vi "CRYSmoothing Waveform.vi"(8 "Weight Mode":u16(ring) items=["None", "Hanning"], 9 "Width (s)":dbl, 11 "Wave In":T1={"Waveform"={"X0"=0.0, "dX"=0.0, "Y"=[]}, "X data"=1, "Y data"=1, "Y axis"=1, "X unit"="s", "Y unit"="V", "Y dB ref"=1.0, "display Y"=TRUE, "display X"=TRUE, "Overload?"=FALSE, "Test Info"="", "Step No."=0, "Name"="", "protected"=FALSE, "Sqc history"=[], "Signal Channel ID"=0, "Plot Settings"={"Color"=0, "Interpolation"=0, "Point Style"=0, "Line Style"=0, "Point Color"=0, "Line Width"=0, "Bar Plot Style"=0, "Fill To"=0}, "AutoProtect"=FALSE} {"Y dB ref" format="%.1f"; "Y axis" items=["Log", "Lin"]; "Y data" items=["dB", "Lin"]; "X data" items=["dB", "Lin"]}) -> (3 "Wave out":T1={"Waveform"={"X0"=0.0, "dX"=0.0, "Y"=[]}, "X data"=1, "Y data"=1, "Y axis"=1, "X unit"="s", "Y unit"="V", "Y dB ref"=1.0, "display Y"=TRUE, "display X"=TRUE, "Overload?"=FALSE, "Test Info"="", "Step No."=0, "Name"="", "protected"=FALSE, "Sqc history"=[], "Signal Channel ID"=0, "Plot Settings"={"Color"=0, "Interpolation"=0, "Point Style"=0, "Line Style"=0, "Point Color"=0, "Line Width"=0, "Bar Plot Style"=0, "Fill To"=0}, "AutoProtect"=FALSE} {"Y dB ref" format="%.1f"; "Y axis" items=["Log", "Lin"]; "Y data" items=["dB", "Lin"]; "X data" items=["dB", "Lin"]})   [LabVIEW 2013]
uses:
  Typedef Control/CRYWaveform Cluster.ctl
  <vilib>/Analysis/2dsp.llb/1D Convolution (DBL).vi
  <vilib>/Analysis/0measdsp.llb/Scaled Time Domain Window (DBL).vi
  <vilib>/Analysis/NI_AALPro.lvlib
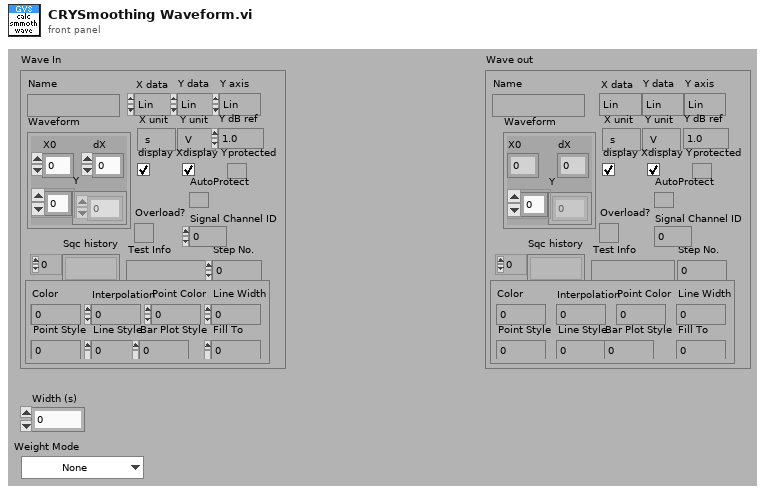
[diagram p1: front panel]
types:
  T1 = typedef "CRYWaveform Cluster.ctl" = cluster{"Waveform":cluster{"X0":dbl, "dX":dbl, "Y":sgl[]}, "X data":u16, "Y data":u16, "Y axis":u16, "X unit":string, "Y unit":string, "Y dB ref":dbl, "display Y":bool, "display X":bool, "Overload?":bool, "Test Info":string, "Step No.":i32, "Name":string, "protected":bool, "Sqc history":string[], "Signal Channel ID":i32, "Plot Settings":cluster{"Color":u32, "Interpolation":u8, "Point Style":u8, "Line Style":u8, "Point Color":u32, "Line Width":u8, "Bar Plot Style":u8, "Fill To":i16}, "AutoProtect":bool}
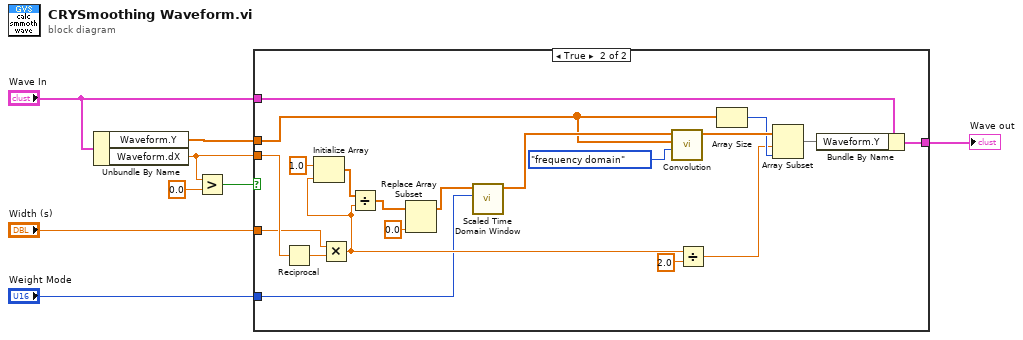
[diagram p0: block diagram]
diagram:
  n1 = Unbundle By Name("Wave In") -> ("Waveform.Y"=w8:sgl[], "Waveform.dX"=w1:dbl)
  n2 = Greater?(x=w1, y=0.0) -> (0:w2:bool)
  n3 = case shown="True" w2 {
    tunnel: w8 -> [_ w17]
    tunnel: w1 -> [_ w15]
    tunnel: "Wave In" -> [w9 w13]
    tunnel: "Width (s)" -> [_ w12]
    tunnel: "Weight Mode" -> [_ w11]
    tunnel: [w9 w10] -> w4
    frame False {
    }
    frame True {
      n4 = Reciprocal(x=w15) -> (1/x=w14:dbl)
      n5 = Multiply(x=w12, y=w14) -> (x*y=w20:dbl)
      n6 = Initialize Array(1.0 ("element"), w20) -> (w28:dbl[])
      n7 = Divide(x=w28, y=w20) -> (x/y=w25:dbl[])
      n8 = Replace Array Subset(array=w25, new element=0.0 ("new element/subarray")) -> (w26:dbl[])  [unwired: 1 in]
      n9 = call-poly <vilib>:"Scaled Time Domain Window.vi"("window"=w11, "X"=w26) -> ("Windowed X"=w22:dbl[])  [unwired: 7 in, 2 out]
      n10 = call-poly <vilib>:"Convolution.vi"("algorithm"=enum32{"direct", "frequency domain"}."frequency domain", "Y"=w17, "X"=w22) -> ("X * Y"=w23:dbl[])  [unwired: 7 in, 1 out]
      n11 = Divide(x=w20, y=2.0) -> (x/y=w18:dbl)
      n12 = Array Size(array=w17) -> (size(s)=w21:i32)
      n13 = Array Subset(array=w23, index=w18, length=w21) -> (w16:dbl[])
      n14 = Bundle By Name(cluster=w13, "Waveform.Y"=w16) -> (w10:T1)
    }
  }
  "Wave out" <- w4
